vi "AddAdditionalNewPage.vi"(8 "Fehler (Eingang, kein Fehler)":errorcluster, 11 "Context (Eingang)":refnum<class "Context.lvclass">) -> (0 "Fehler (Ausgang)":errorcluster, 3 "Context Out":refnum<class "Context.lvclass">)   [LabVIEW 2020, in "PDF Interface.lvlib"]
doc: "To add an addiotional Page to an (or more) already existing pages within the PDF."
uses:
  PDF Interface.lvlib
  <vilib>/Simplicity AI/SAI_PDF_API/Classes/Context/Context.lvclass
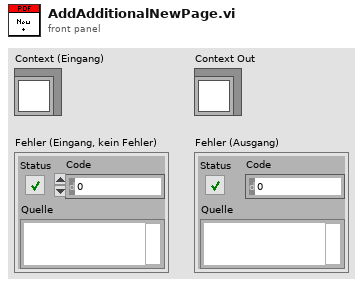
[diagram p1: front panel]
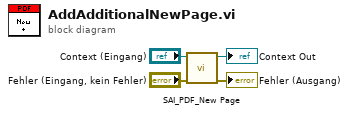
[diagram p0: block diagram]
diagram:
  n1 = call <vilib>:"SAI_PDF_New Page.vi"("error in"="Fehler (Eingang, kein Fehler)", "Context In"="Context (Eingang)") -> ("error out"=→"Fehler (Ausgang)":errorcluster, "Context Out"=→"Context Out":refnum<class "Context.lvclass">)  [unwired: 8 in]
